vi "TestFlowID - Write.vi"(8 "error in (no error)":errorcluster, 10 "TestFlowID":string, 11 "Globals in":refnum<class "TSM Context Data Access.lvclass">) -> (0 "error out":errorcluster, 3 "Globals out":refnum<class "TSM Context Data Access.lvclass">)   [LabVIEW 2019, in "TSM Context Data Access.lvclass"]
uses:
  TSM Context Data Access.lvclass
  TSM Context Data Access.lvclass/TSM Context Data Access.ctl
  <vilib>/NI_TestStand_SemiconductorModule/NI_TestStand_Semiconductor_Module.lvlibp
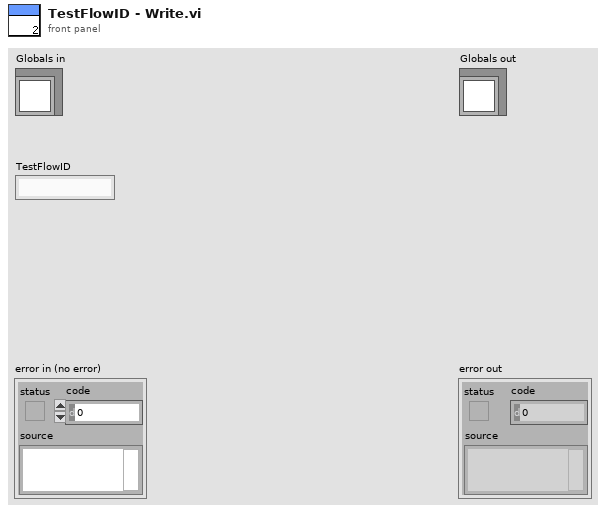
[diagram p1: front panel]
types:
  T1 = typedef "NI_TestStand_Semiconductor_Module.lvlibp/SemiconductorModuleContext.ctl" = refnum<k7>
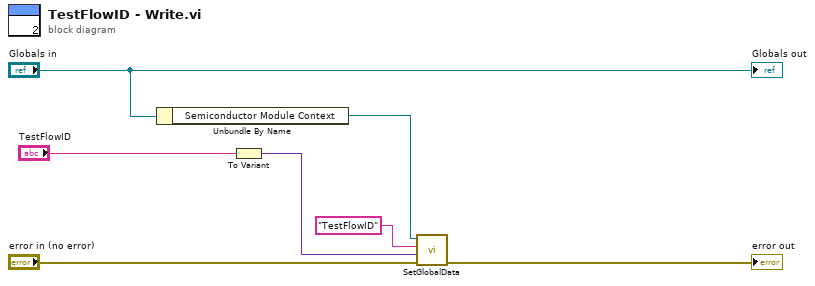
[diagram p0: block diagram]
diagram:
  n1 = Unbundle By Name("Globals in") -> ("Semiconductor Module Context"=w1:T1)
  n2 = To Variant(anything="TestFlowID") -> (Variant=w4:variant)
  n3 = call <vilib>:"SetGlobalData.vi"("error in (no error)"="error in (no error)", "Data"=w4, "Data Id"="TestFlowID", "Semiconductor Module Context"=w1) -> ("error out"=→"error out":errorcluster)  [unwired: 5 in, 1 out]
  "Globals out" <- "Globals in"
